vi "SwitchedACIR.vi"(4 "ACIR ClassName":string="Sim ACIR\\Sim ACIR.lvclass", 5 "Setting":T1={"Freq"=1000.0, "Range"=enum."10m Ohm", "Measurements"=enum."OCV"} {"Freq" min=0.1 max=1050.0 step=0.01 format="%_5e"}, 6 "ACIR Ref":string, 7 "Connection(s)":string="102", 8 "error in":errorcluster, 9 "Switch Ref":string, 10 "Switch ClassName":string="Sim Switch\\Sim Switch.lvclass", 11 "Base Path":path=path "C:/GitHub/OOP Template/HAL/Concrete") -> (0 "error out":errorcluster, 3 "Measurements":dbl=0.0001541850001696224)   [LabVIEW 2019, in "MAL.lvlib"]
uses:
  MAL.lvlib
  Hardware Abstraction/Harware Abstraction/Switch/Switch.lvclass
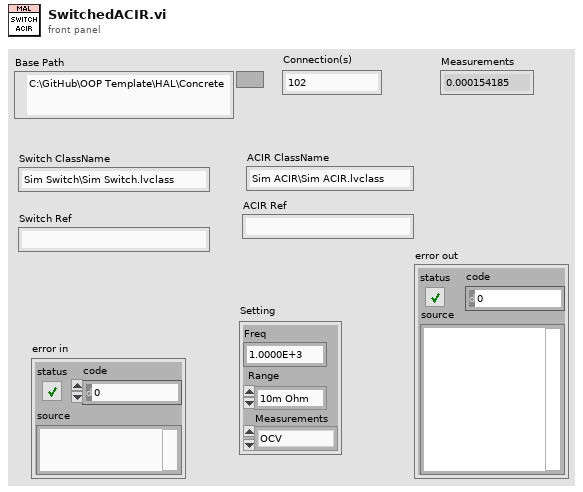
[diagram p1: front panel]
types:
  T1 = cluster{"Freq":dbl, "Range":enum16{"3m Ohm", "10m Ohm", "100m Ohm"}, "Measurements":enum16{"Impedence", "Phase Angle", "OCV"}}
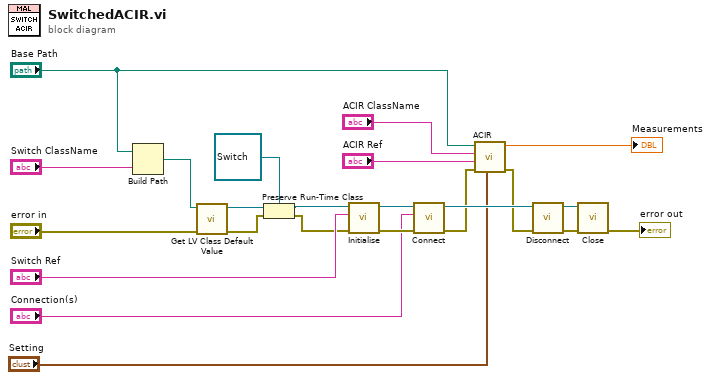
[diagram p0: block diagram]
diagram:
  n1 = Build Path(base path="Base Path", name or relative path="Switch ClassName") -> (appended path=w4:path)
  n2 = call <vilib>:"Get LV Class Default Value.vi"("error in (no error)"="error in", "class path"=w4) -> ("error out"=w21:errorcluster, "object"=w22:refnum<class>)  [unwired: 8 in]
  n3 = Preserve Run-Time Class(object in=w22, error in=w21, 2:refnum<class "Switch.lvclass"> refnum ("Hardware Abstration.lvlib:Switch.lvclass")) -> (object out=w19:refnum<class "Switch.lvclass">, error out=w18:errorcluster)
  n4 = call-dynamic "Initialise.vi"("error in (no error)"=w18, "Instrument Ref"="Switch Ref", "Instrument in"=w19) -> ("error out"=w16:errorcluster, "Instrument out"=w15:refnum<class "Switch.lvclass">)  [unwired: 7 in]
  n5 = call-dynamic "Connect.vi"("error in (no error)"=w16, "Channel(s)"="Connection(s)", "Switch in"=w15) -> ("error out"=w10:errorcluster, "Switch out"=w11:refnum<class "Switch.lvclass">)  [unwired: 7 in]
  n6 = call "ACIR.vi"("Setting"="Setting", "error in"=w10, "ACIR Ref"="ACIR Ref", "ACIR Class"="ACIR ClassName", "Base Path"="Base Path") -> ("error out"=w9:errorcluster, "Measurements"=→"Measurements":dbl)  [unwired: 5 in]
  n7 = call-dynamic "Disconnect.vi"("error in (no error)"=w9, "Switch in"=w11) -> ("error out"=w14:errorcluster, "Switch out"=w13:refnum<class "Switch.lvclass">)  [unwired: 8 in]
  n8 = call-dynamic "Close.vi"("error in (no error)"=w14, "Instrument in"=w13) -> ("error out"=→"error out":errorcluster)  [unwired: 8 in, 1 out]
